vi "结果查询.vi"() -> ()   [LabVIEW 2013]
panel:
  out "添加的数组":string[][](array[string])
  out "数组 3":cluster{"字符串":i32, i32}[](array[cluster])
  out "数组 2":cluster{"字符串":i32, i32}[](array[cluster])
  in  "connection information 2":path
  in  "返回":bool
  in  "生成报表":bool
  in  "簇":T1
  out "年龄":string
  out "性别":string
  out "姓名":string
  in  "身份证输入框":string(combo)
  in  "查询":bool
  # "结果查询"
  # "身份证号码"
  # "姓名"
  # "性别"
  # "年龄"
  # "500"
  # "1000"
  # "250"
  # "左耳测评结果"
  # "筛查频点(Hz)"
  # "左耳听阈（dB）"
  # "右耳听阈（dB）"
  # "右耳测评结果"
  # "语音测评准确率"
  # "问卷调查"
  # "dB"
  # "Hz"
  # "dB"
  # "Hz"
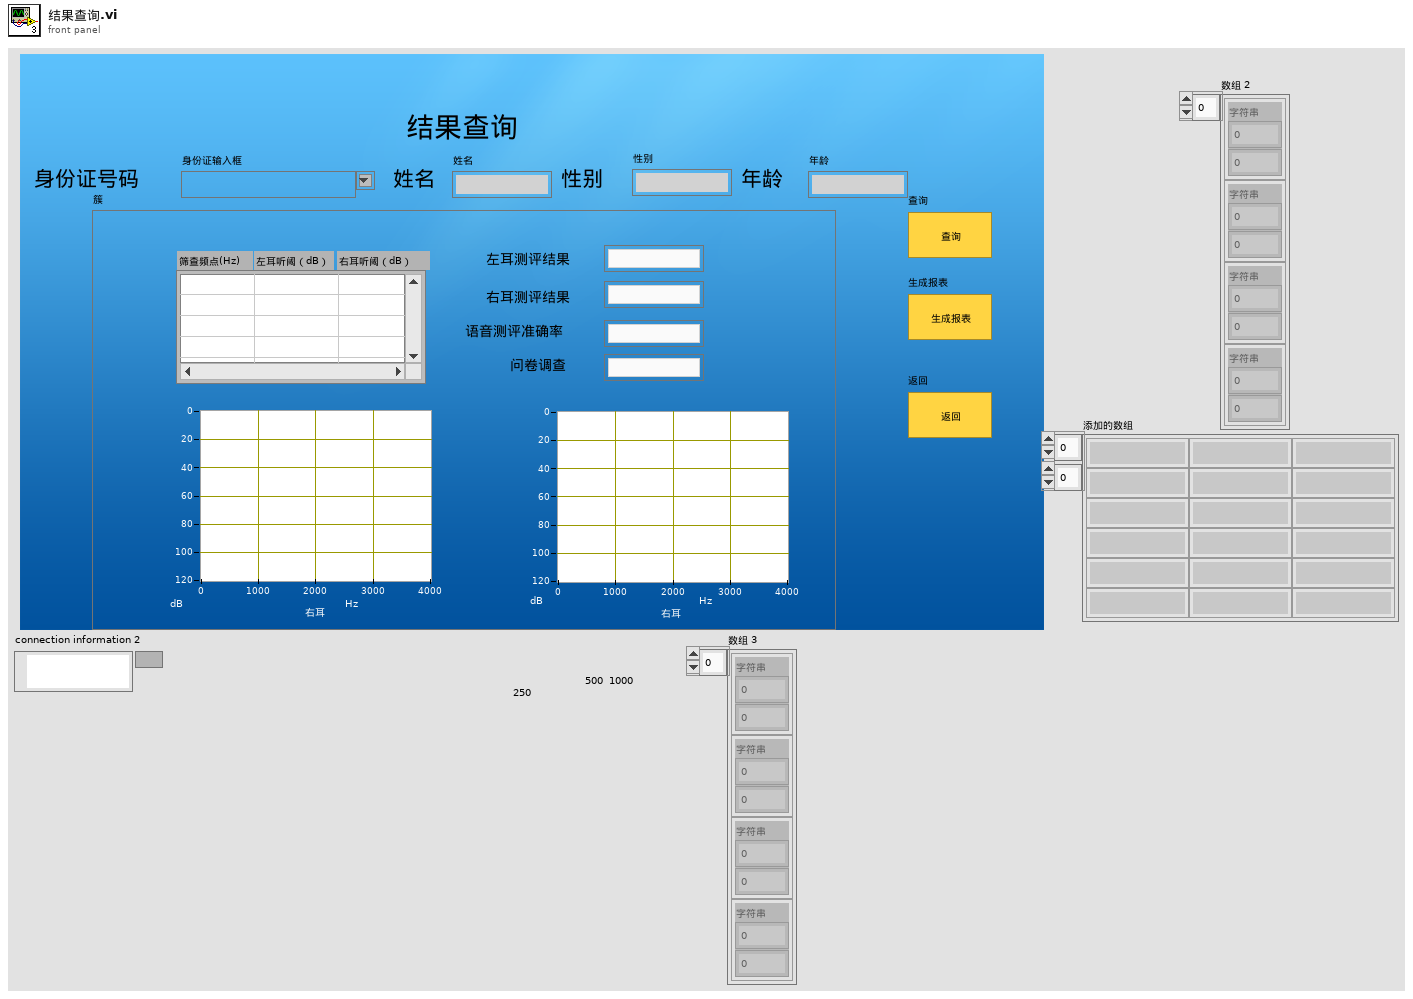
[diagram p1: front panel]
types:
  T1 = cluster{"波形图表 2":cluster{"X":dbl, "Y":dbl}[], "波形图表 3":cluster{"X":dbl, "Y":dbl}[], "左耳测评结果":string, "右耳测评结果":string, "语音测评结果":string, "问卷调查":string, "数据":string[][]}
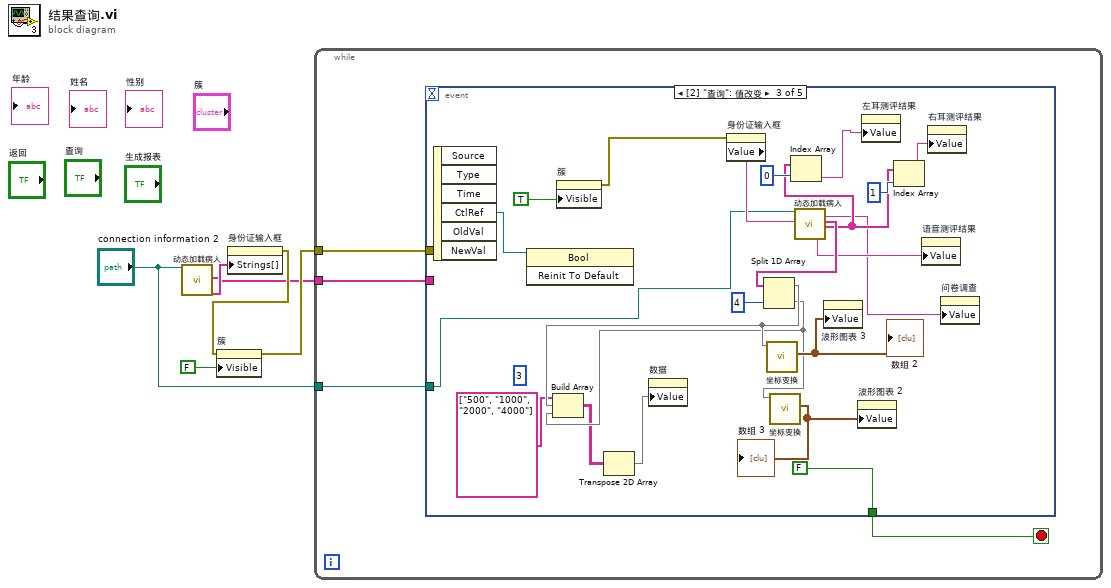
[diagram p0: block diagram]
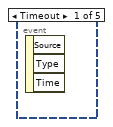
[diagram p2: hidden frame]
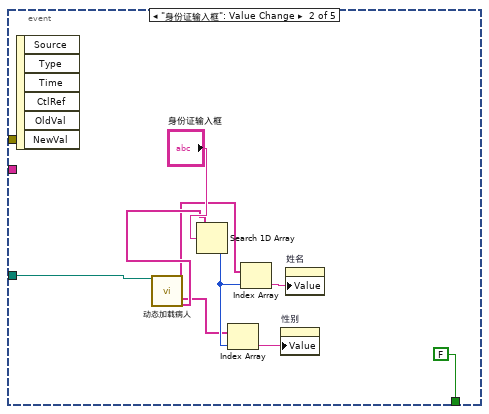
[diagram p3: hidden frame]
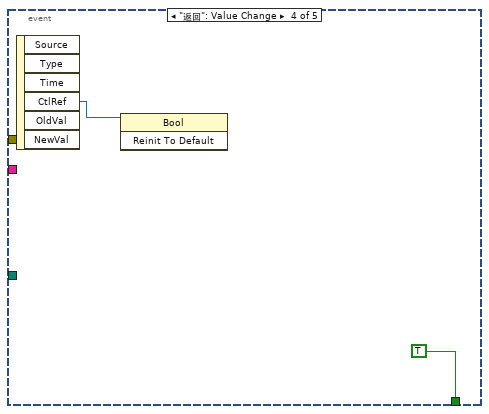
[diagram p4: hidden frame]
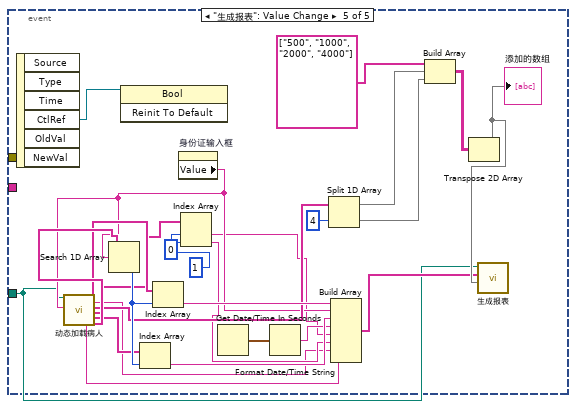
[diagram p5: hidden frame]
diagram:
  n1 = call "动态加载病人.vi"("connection information 2"="connection information 2") -> ("快速测查数据"=w1:string[], "身份证"=w6:string[])  [unwired: 12 in, 5 out]
  n2 = property on="身份证输入框" class="CmbBox"("Strings[]"=w6) -> (error out=w5:errorcluster)  [unwired: 2 in, 1 out]
  n3 = property on="簇" class="Clust (严格)"(error in=w5, "Visible"=FALSE) -> (error out=w4:errorcluster)  [unwired: 1 in, 1 out]
  n4 = while {
    tunnel: w4 -> [w10]
    tunnel: "connection information 2" -> [w8]
    tunnel: w1 -> [w7]
    stop <- w9 stop-if-true
    n5 = event shown="[2] \"查询\": 值改变" {
      selector: _ -> [_ _ _ _ _]
      dyn-events: _ -> [_ _ _ _ _]
      timeout: _ -> [_ _ _ _ _]
      tunnel: w10 -> [_ _ _ _ _]
      tunnel: [_ FALSE FALSE TRUE _] -> w9
      tunnel: w8 -> [_ w11 w29 _ w44]
      tunnel: w7 -> [_ _ _ _ _]
      event Timeout {
        n6 = event-data() -> ()  [unwired: 1 in, 3 out]
      }
      event "身份证输入框": Value Change {
        n7 = event-data() -> ()  [unwired: 1 in, 6 out]
        n8 = call "动态加载病人.vi"("connection information 2"=w11) -> ("姓名"=w14:string[], "性别"=w16:string[], "身份证"=w17:string[])  [unwired: 12 in, 4 out]
        n9 = Search 1D Array(1D array=w17, element="身份证输入框") -> (index of element=w18:i32)  [unwired: 1 in]
        n10 = Index Array(array=w16, index=w18) -> (element=w15:string)
        n11 = Index Array(array=w14, index=w18) -> (element=w13:string)
        n12 = property on="性别" class="Str"("Value"=w15) -> ()  [unwired: 2 in, 2 out]
        n13 = property on="姓名" class="Str"("Value"=w13) -> ()  [unwired: 2 in, 2 out]
      }
      event "查询": Value Change {
        (unwired) 3
        n14 = event-data() -> ("CtlRef"=w38:refnum<vi>)  [unwired: 1 in, 5 out]
        n15 = invoke class="Bool" method="Reinit To Default"(reference=w38) -> ()  [unwired: 2 in, 3 out]
        n16 = property on="簇" class="Clust (严格)"("Visible"=TRUE) -> (error out=w28:errorcluster)  [unwired: 2 in, 1 out]
        n17 = property on="身份证输入框" class="CmbBox"(error in=w28) -> ("Value"=w41:string)  [unwired: 1 in, 2 out]
        n18 = call "动态加载病人.vi"("connection information 2"=w29, "输入身份证"=w41) -> ("语音测评"=w26:string, "问卷调查"=w25:string, "快速测查数据"=w32:string[], "左右耳结论"=w27:string[])  [unwired: 11 in, 3 out]
        n19 = Split 1D Array(array=w32, index=4) -> (first subarray=w24:string[], second subarray=w23:string[])
        n20 = Build Array(string[] ["500", "1000", "2000", "4000"], w24, w23) -> (w21:string[][])
        n21 = Transpose 2D Array(2D array=w21) -> (transposed array=w20:string[][])
        n22 = property on="数据" class="Tbl (严格)"("Value"=w20) -> ()  [unwired: 2 in, 2 out]
        n23 = call "坐标变换.vi"("数组"=w24) -> ("数组 2"=w35:cluster{"字符串":i32, i32}[])  [unwired: 10 in]
        "数组 2" <- w35
        n24 = call "坐标变换.vi"("数组"=w23) -> ("数组 2"=w36:cluster{"字符串":i32, i32}[])  [unwired: 10 in]
        "数组 3" <- w36
        n25 = Index Array(array=w27, index=0) -> (element=w33:string)
        n26 = property on="波形图表 3" class="XYGraph (严格)"("Value"=w35) -> ()  [unwired: 2 in, 2 out]
        n27 = property on="波形图表 2" class="XYGraph (严格)"("Value"=w36) -> ()  [unwired: 2 in, 2 out]
        n28 = property on="左耳测评结果" class="Str"("Value"=w33) -> ()  [unwired: 2 in, 2 out]
        n29 = Index Array(array=w27, index=1) -> (element=w30:string)
        n30 = property on="语音测评结果" class="Str"("Value"=w26) -> ()  [unwired: 2 in, 2 out]
        n31 = property on="右耳测评结果" class="Str"("Value"=w30) -> ()  [unwired: 2 in, 2 out]
        n32 = property on="问卷调查" class="Str"("Value"=w25) -> ()  [unwired: 2 in, 2 out]
      }
      event "返回": Value Change {
        n33 = event-data() -> ("CtlRef"=w42:refnum<vi>)  [unwired: 1 in, 5 out]
        n34 = invoke class="Bool" method="Reinit To Default"(reference=w42) -> ()  [unwired: 2 in, 3 out]
      }
      event "生成报表": Value Change {
        n35 = event-data() -> ("CtlRef"=w69:refnum<vi>)  [unwired: 1 in, 5 out]
        n36 = invoke class="Bool" method="Reinit To Default"(reference=w69) -> ()  [unwired: 2 in, 3 out]
        n37 = property on="身份证输入框" class="CmbBox"() -> ("Value"=w52:string)  [unwired: 2 in, 2 out]
        n38 = call "动态加载病人.vi"("connection information 2"=w44, "输入身份证"=w52) -> ("语音测评"=w46:string, "姓名"=w61:string[], "问卷调查"=w47:string, "快速测查数据"=w55:string[], "左右耳结论"=w56:string[], "性别"=w62:string[], "身份证"=w63:string[])  [unwired: 11 in]
        n39 = Search 1D Array(1D array=w63, element=w52) -> (index of element=w64:i32)  [unwired: 1 in]
        n40 = Index Array(array=w62, index=w64) -> (element=w59:string)
        n41 = Index Array(array=w61, index=w64) -> (element=w60:string)
        n42 = Index Array(array=w56, index #1=0, index #2=1) -> (element #1=w49:string, element #2=w48:string)
        n43 = Get Date/Time In Seconds() -> (seconds since 1Jan1904=w58:timestamp)
        n44 = Format Date/Time String(seconds (now)=w58) -> (date/time string=w57:string)  [unwired: 2 in]
        n45 = Split 1D Array(array=w55, index=4) -> (first subarray=w54:string[], second subarray=w53:string[])
        n46 = Build Array(w60, w52, w59, w57, w49, w48, w47, w46) -> (w45:string[])
        n47 = Build Array(string[] ["500", "1000", "2000", "4000"], w54, w53) -> (w66:string[][])
        n48 = Transpose 2D Array(2D array=w66) -> (transposed array=w65:string[][])
        "添加的数组" <- w65
        n49 = call "生成报表.vi"("template (empty)"=w44, "测试结果"=w45, "左右耳数据"=w65) -> ()  [unwired: 6 in]
      }
    }
  }
